vi "Main.vi"() -> ()   [LabVIEW 2015]
uses:
  TypeDefs/Queue Data.ctl
  SubVIs/App Data.vi
  SubVIs/App Strings.vi
  FGV/Timer Actions.ctl
panel:
  in  "Period [s]":dbl
  in  "Device name":tag="myDAQ1"
  out "Time Elapsed":dbl format="%<%M:%S>t"
  out "Status":string
  in  "Time [ms]":dbl
  in  "Frequency":dbl
  in  "Stop Button":bool
  in  "Acquire Button":bool
  out "Waveform Graph":dbl[](graph)
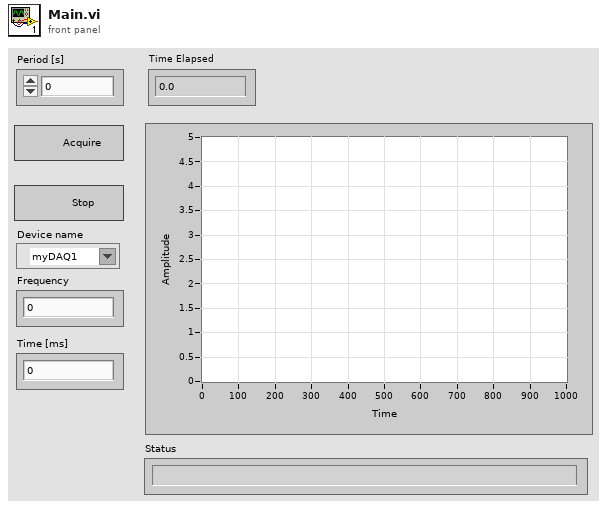
[diagram p1: front panel]
types:
  T1 = typedef "Timer Actions.ctl" = enum16{"Reset", "Get"}
  T2 = typedef "Queue Data.ctl" = cluster{"Action":string}
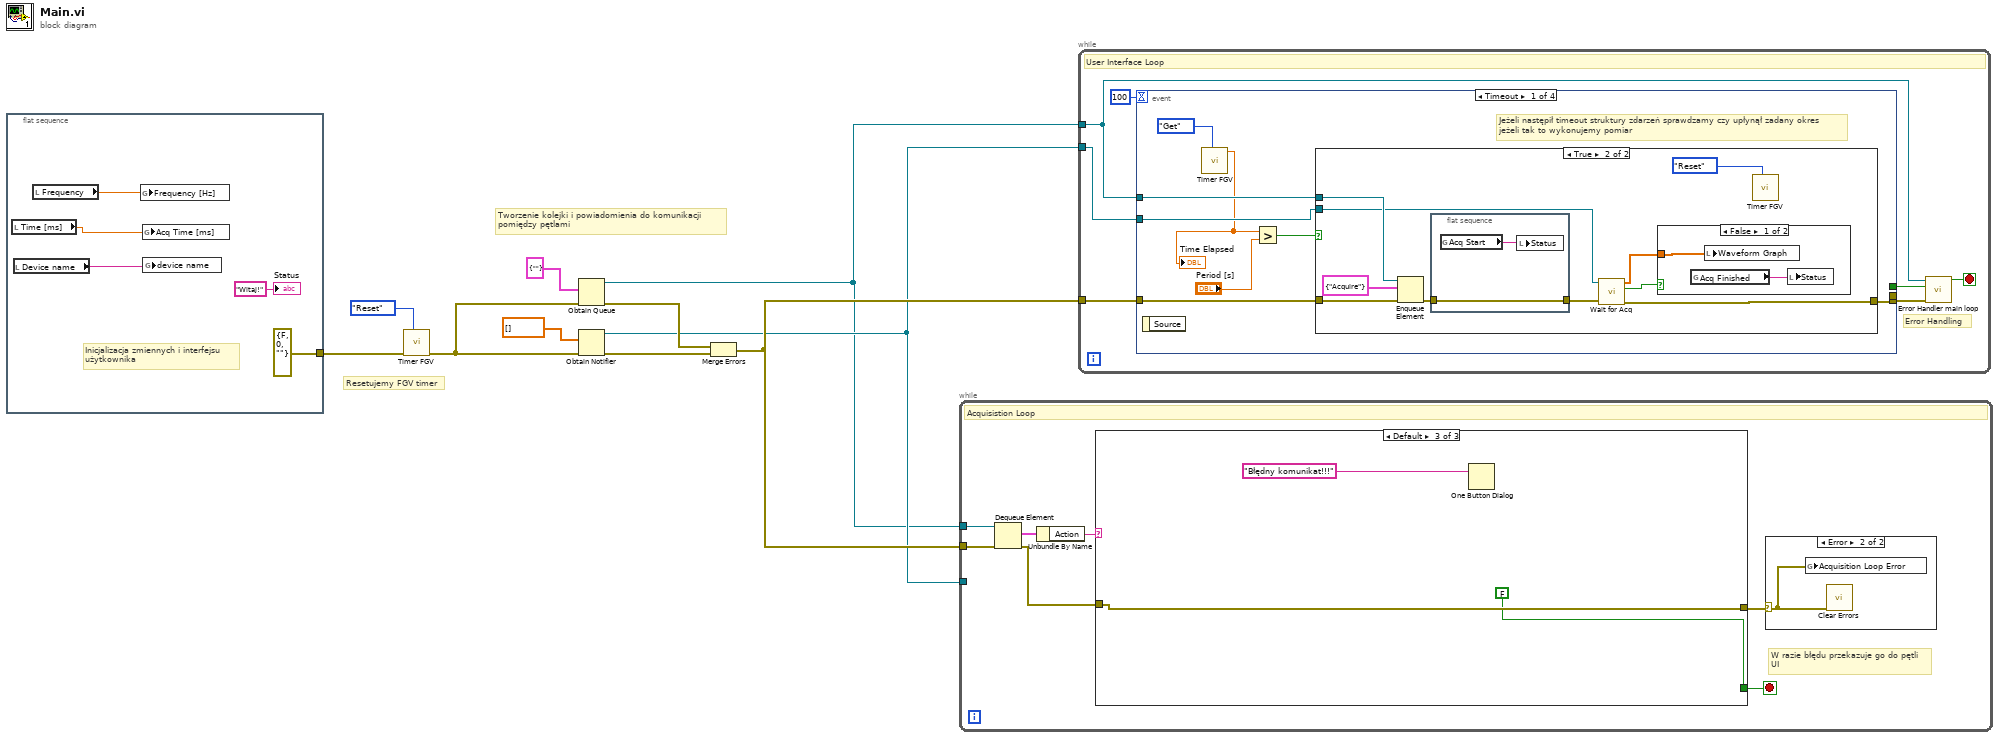
[diagram p0: block diagram]
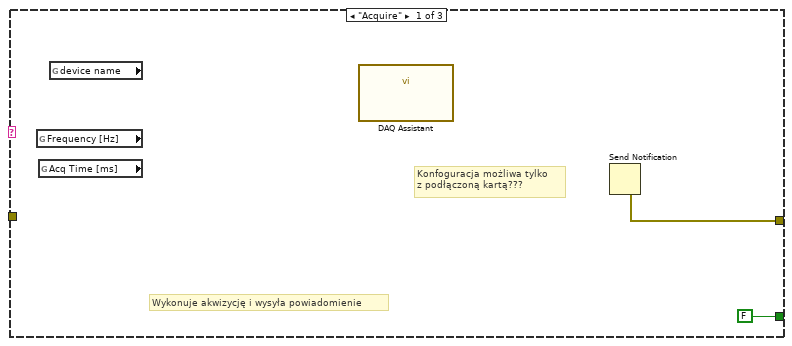
[diagram p3: hidden frame]
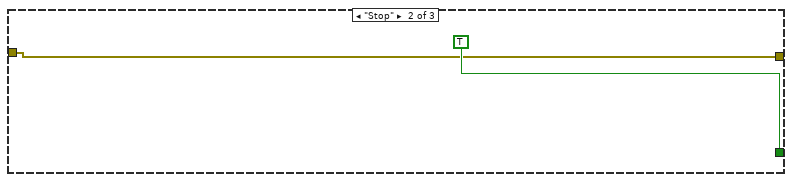
[diagram p4: hidden frame]
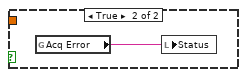
[diagram p6: hidden frame]
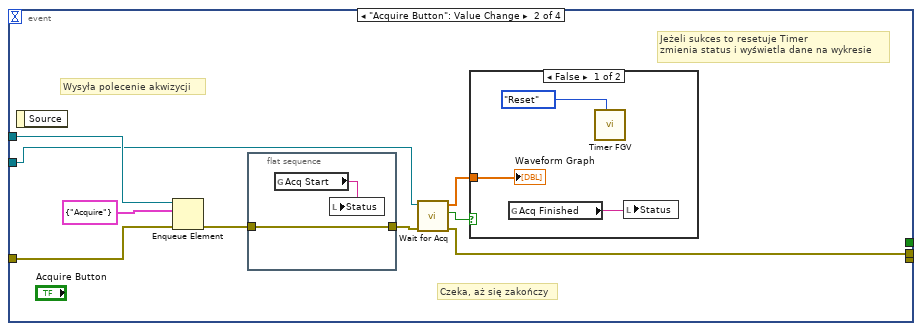
[diagram p7: hidden frame]
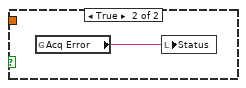
[diagram p8: hidden frame]
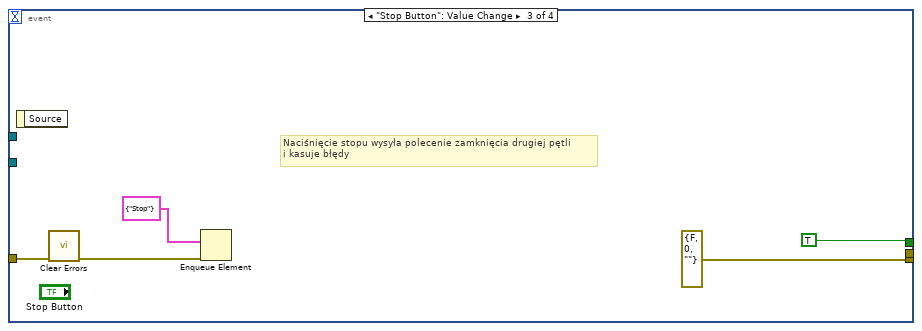
[diagram p9: hidden frame]
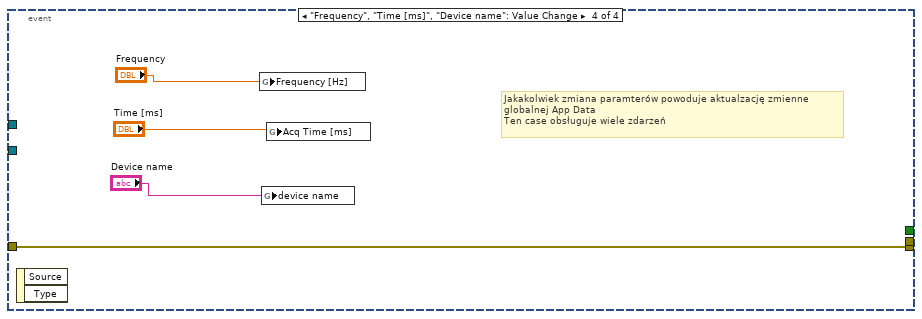
[diagram p10: hidden frame]
diagram:
  # "Resetujemy FGV timer"
  # "Tworzenie kolejki i powiadomienia do komunikacji \npomiędzy pętlami"
  n1 = flat-sequence {
    tunnel: [errorcluster {"status"=FALSE, "code"=0, "source"=""} ("error constant")] -> w3
    frame #0 {
      # "Inicjalizacja zmiennych i interfejsu \nużytkownika"
      n2 = local read "Time [ms]"() -> (w12:dbl)
      n3 = local read "Device name"() -> (w11:tag)
      n4 = local read "Frequency"() -> (w13:dbl)
      n5 = global write "App Data.vi" "Frequency [Hz]"(w13) -> ()
      n6 = global write "App Data.vi" "Acq Time [ms]"(w12) -> ()
      n7 = global write "App Data.vi" "device name"(w11) -> ()
      "Status" <- "Witaj!" ("Status")
    }
  }
  n8 = call "Timer FGV.vi"("Action"=Timer_Actions."Reset", "error in (no error)"=w3) -> ("error out"=w2:errorcluster)  [unwired: 8 in, 1 out]
  n9 = Obtain Queue(element data type=T2 {"Action"=""}, error in (no error)=w2) -> (queue out=w4:refnum<queue>, error out=w9:errorcluster)  [unwired: 3 in, 1 out]
  n10 = Obtain Notifier(notification data type=dbl[] [], error in (no error)=w2) -> (notifier out=w5:refnum<notifier>, error out=w7:errorcluster)  [unwired: 2 in, 1 out]
  n11 = Merge Errors(w9, w7) -> (w6:errorcluster)
  n12 = while {
    tunnel: w6 -> [w20]
    tunnel: w4 -> [w19]
    tunnel: w5 -> [_]
    stop <- w17 stop-if-true
    # "W razie błędu przekazuje go do pętli\nUI"
    # "Acquisistion Loop"
    n13 = Dequeue Element(queue=w19, error in (no error)=w20) -> (element=w22:T2, error out=w18:errorcluster)  [unwired: 1 in, 2 out]
    n14 = Unbundle By Name(w22) -> ("Action"=w21:string)
    n15 = case shown="Default" w21 {
      tunnel: w18 -> [_ w26 w29]
      tunnel: [FALSE TRUE FALSE] -> w17
      tunnel: [w24 w26 w29] -> w16
      frame "Acquire" {
        # "Konfoguracja możliwa tylko\nz podłączoną kartą???"
        # "Wykonuje akwizycję i wysyła powiadomienie"
        n16 = global read "App Data.vi" "Frequency [Hz]"() -> ()  [unwired: 1 out]
        n17 = global read "App Data.vi" "Acq Time [ms]"() -> ()  [unwired: 1 out]
        n18 = global read "App Data.vi" "device name"() -> ()  [unwired: 1 out]
        n19 = call "DAQ Assistant"() -> ()  [unwired: 12 in]
        n20 = Send Notification() -> (error out=w24:errorcluster)  [unwired: 3 in, 1 out]
      }
      frame "Stop" {
      }
      frame Default {
        n21 = One Button Dialog(message="Błędny komunikat!!!") -> ()  [unwired: 1 in, 1 out]
      }
    }
    n22 = case shown="Error" w16 {
      selector: w16 -> [_ w23]
      frame No Error {
      }
      frame Error {
        n23 = global write "App Data.vi" "Acquisition Loop Error"(w23) -> ()
        n24 = call <vilib>:"Clear Errors.vi"("error in (no error)"=w23) -> ()  [unwired: 5 in, 2 out]
      }
    }
  }
  n25 = while {
    tunnel: w6 -> [w36]
    tunnel: w4 -> [w32]
    tunnel: w5 -> [w31]
    stop <- w33 stop-if-true
    # "Error Handling"
    # "User Interface Loop"
    n26 = event shown="[0] Timeout" {
      selector: _ -> [_ _ _ _]
      dyn-events: _ -> [_ _ _ _]
      timeout: 100 -> [_ _ _ _]
      tunnel: w36 -> [w43 w68 w78 w85]
      tunnel: [w42 _ errorcluster {"status"=FALSE, "code"=0, "source"=""} ("error constant") w85] -> w34
      tunnel: [_ _ TRUE _] -> w35
      tunnel: w32 -> [w41 w69 _ _]
      tunnel: w31 -> [w40 w62 _ _]
      tunnel: [_ w65 _ _] -> _
      event Timeout {
        # "Jeżeli następił timeout struktury zdarzeń sprawdzamy czy upłynął zadany okres \njeżeli tak to wykonujemy pomiar"
        n27 = event-data() -> ()  [unwired: 1 in, 1 out]
        n28 = call "Timer FGV.vi"("Action"=Timer_Actions."Get") -> ("Elapsed Time"=w38:dbl)  [unwired: 9 in, 1 out]
        "Time Elapsed" <- w38
        n29 = Greater?(x=w38, y="Period [s]") -> (0:w44:bool)
        n30 = case shown="True" w44 {
          tunnel: w43 -> [w46 w56]
          tunnel: [w46 w49] -> w42
          tunnel: w41 -> [_ w48]
          tunnel: w40 -> [_ w47]
          frame False {
          }
          frame True {
            n31 = Enqueue Element(queue=w48, element=T2 {"Action"="Acquire"}, error in (no error)=w56) -> (error out=w54:errorcluster)  [unwired: 1 in, 2 out]
            n32 = flat-sequence {
              tunnel: w54 -> [w60]
              tunnel: [w60] -> w53
              frame #0 {
                n33 = global read "App Strings.vi" "Acq Start"() -> (w61:string)
                n34 = local write "Status"(w61) -> ()
              }
            }
            n35 = call "Wait for Acq.vi"("error in (no error)"=w53, "Notifier in"=w47) -> ("error out"=w49:errorcluster, "timed out?"=w50:bool, "Array"=w52:dbl[])  [unwired: 7 in]
            n36 = case shown="False" w50 {
              tunnel: w52 -> [w57 _]
              frame False {
                n37 = global read "App Strings.vi" "Acq Finished"() -> (w58:string)
                n38 = local write "Waveform Graph"(w57) -> ()
                n39 = local write "Status"(w58) -> ()
              }
              frame True {
                n40 = global read "App Strings.vi" "Acq Error"() -> (w59:string)
                n41 = local write "Status"(w59) -> ()
              }
            }
            n42 = call "Timer FGV.vi"("Action"=Timer_Actions."Reset") -> ()  [unwired: 9 in, 2 out]
          }
        }
      }
      event "Acquire Button": Value Change {
        # "Jeżeli sukces to resetuje Timer\nzmienia status i wyświetla dane na wykresie"
        # "Czeka, aż się zakończy"
        # "Wysyła polecenie akwizycji"
        n43 = event-data() -> ()  [unwired: 1 in, 1 out]
        n44 = Enqueue Element(queue=w69, element=T2 {"Action"="Acquire"}, error in (no error)=w68) -> (error out=w66:errorcluster)  [unwired: 1 in, 2 out]
        n45 = flat-sequence {
          tunnel: [w72] -> w67
          tunnel: w66 -> [w72]
          frame #0 {
            n46 = global read "App Strings.vi" "Acq Start"() -> (w71:string)
            n47 = local write "Status"(w71) -> ()
          }
        }
        n48 = call "Wait for Acq.vi"("error in (no error)"=w67, "Notifier in"=w62) -> ("error out"=w65:errorcluster, "timed out?"=w64:bool, "Array"=w63:dbl[])  [unwired: 7 in]
        n49 = case shown="False" w64 {
          tunnel: w63 -> [w73 _]
          frame False {
            n50 = global read "App Strings.vi" "Acq Finished"() -> (w75:string)
            n51 = call "Timer FGV.vi"("Action"=Timer_Actions."Reset") -> ()  [unwired: 9 in, 2 out]
            n52 = local write "Status"(w75) -> ()
            "Waveform Graph" <- w73
          }
          frame True {
            n53 = global read "App Strings.vi" "Acq Error"() -> (w76:string)
            n54 = local write "Status"(w76) -> ()
          }
        }
      }
      event "Stop Button": Value Change {
        # "Naciśnięcie stopu wysyła polecenie zamknięcia drugiej pętli\ni kasuje błędy"
        n55 = event-data() -> ()  [unwired: 1 in, 1 out]
        n56 = call <vilib>:"Clear Errors.vi"("error in (no error)"=w78) -> ("error out"=w77:errorcluster)  [unwired: 5 in, 1 out]
        n57 = Enqueue Element(element=T2 {"Action"="Stop"}, error in (no error)=w77) -> ()  [unwired: 2 in, 3 out]
      }
      event "Frequency", "Time [ms]", "Device name": Value Change {
        # "Jakakolwiek zmiana paramterów powoduje aktualzację zmienne \nglobalnej App Data\nTen case obsługuje wiele zdarzeń"
        n58 = event-data() -> ()  [unwired: 1 in, 2 out]
        n59 = global write "App Data.vi" "Frequency [Hz]"("Frequency") -> ()
        n60 = global write "App Data.vi" "device name"("Device name") -> ()
        n61 = global write "App Data.vi" "Acq Time [ms]"("Time [ms]") -> ()
      }
    }
    n62 = call "Error Handler main loop.vi"("error in (no error)"=w34, "Exit?"=w35, "Queue in"=w32) -> ("Exit?"=w33:bool)  [unwired: 8 in]
  }
